vi "RSZVB Get TDIF Phase Imbalance Start Phase.vi"(8 "error in (no error)":errorcluster {"code" format="%.0x"}, 10 "Channel (1)":i32=1, 11 "VISA session":refnum<visa-resource-name>) -> (0 "error out":errorcluster {"code" format="%.0x"}, 2 "Start Phase":dbl format="%^.3e", 3 "dup VISA session":refnum<visa-resource-name>)   [LabVIEW 2011]
doc: "This VI returns the start phase for a phase imbalance sweep, which is equal to the left edge of a Cartesian diagram.\n\nNote(s):\n\n(1) This VI is available only with option R&S ZVA-K6.\n\nRemote-control command(s):\nSOURce<Ch>:TDIF:IMBalance:PHASe:STARt?"
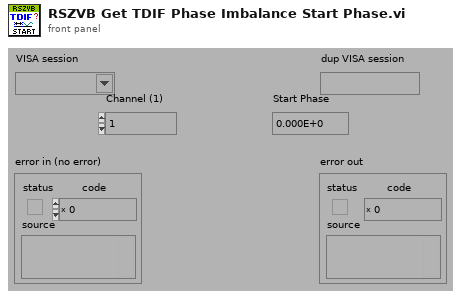
[diagram p1: front panel]
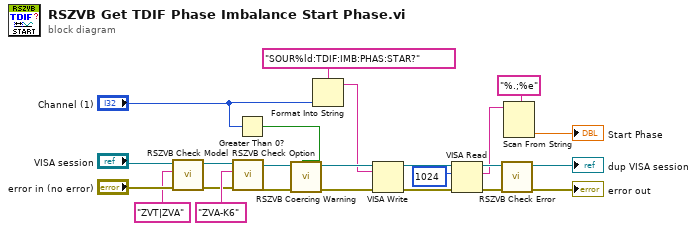
[diagram p0: block diagram]
diagram:
  n1 = call "RSZVB Check Model.vi"("error in (no error)"="error in (no error)", "Model"="ZVT|ZVA" ("Options"), "VISA session"="VISA session") -> ("error out"=w10:errorcluster, "dup VISA session"=w11:refnum<visa-resource-name>)  [unwired: 7 in]
  n2 = call "RSZVB Check Option.vi"("error in (no error)"=w10, "Options"="ZVA-K6", "VISA session"=w11) -> ("error out"=w9:errorcluster, "dup VISA session"=w8:refnum<visa-resource-name>)  [unwired: 7 in]
  n3 = Greater Than 0?(x="Channel (1)") -> (x > 0?=w13:bool)
  n4 = call "RSZVB Coercing Warning.vi"("In Range?"=w13, "error in (no error)"=w9, "VISA session"=w8) -> ("error out"=w16:errorcluster, "dup VISA session"=w17:refnum<visa-resource-name>)  [unwired: 7 in]
  n5 = Format Into String(format string="SOUR%ld:TDIF:IMB:PHAS:STAR?", "Channel (1)") -> (resulting string=w14:string)  [unwired: 2 in, 1 out]
  n6 = VISA Write(VISA resource name=w17, write buffer=w14, error in (no error)=w16) -> (VISA resource name out=w18:refnum<visa-resource-name>, error out=w19:errorcluster)  [unwired: 1 out]
  n7 = VISA Read(VISA resource name=w18, byte count=u32 1024 ("byte count (0)"), error in (no error)=w19) -> (VISA resource name out=w23:refnum<visa-resource-name>, read buffer=w20:string, error out=w22:errorcluster)  [unwired: 1 out]
  n8 = call "RSZVB Check Error.vi"("error in (no error)"=w22, "VISA session"=w23) -> ("error out"=→"error out":errorcluster, "dup VISA session"=→"dup VISA session":refnum<visa-resource-name>)  [unwired: 8 in]
  n9 = Scan From String(format string="%.;%e", input string=w20) -> (output 1=→"Start Phase":dbl)  [unwired: 3 in, 3 out]
